vi "Error Control.vi"(4 "Command":T1, 5 "error in (no error)":errorcluster, 8 "Source":string) -> (0 "error out":errorcluster)   [LabVIEW 2020]
doc: "[Ver 1.00]\nREUSEABLE COMPONENT\nDESCRIPTION\nReuseable Component\nDisplays or logs errors. \n\nCOMMANDS\nNo Command - Error :Throw the error dialog.\nSet to Dev Mode : This should be set first, when Set Error is called the dialog will be displayed. \nSet to Released Mode : This should be set first, when Set Error is called the error will be quietly filed away.\nSet Error : Throw or Log an error.\nLog Error : Log an error regardless of Mode.\nThrow Error : Throw dialog regardless of Mode.\nLog & Throw Error : Do both regardless of Mode.\n\nERROR HANDLING\nWill throw an error if No Command is set\n\n---------------------------------------------------------\nVERSION CONTROL\n1.00 New version SSDC 14/3/2000"
uses:
  Controls/DisplayQCommand.ctl
  Error/ErrorMessage.ctl
  ErrorCommand.ctl
panel:
  # "Input"
  # "Output"
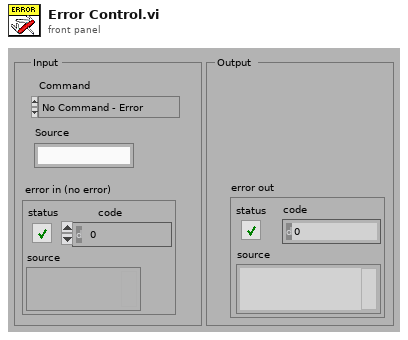
[diagram p1: front panel]
types:
  T1 = typedef "ErrorCommand.ctl" = enum16{"No Command - Error", "Set to Dev Mode", "Set To Released Mode", "Set Error", "Log Error", "Throw Error", "Log & Throw Error", "Set Error Timed"}
  T2 = typedef "ErrorMessage.ctl" = enum16{"No Message - Ignore", "Display Message", "Stop"}
  T3 = typedef "DisplayQCommand.ctl" = enum16{"No Command - Error", "Initialise", "Get Q Reference", "Add Item to Bottom", "Add Item to Top", "Flush Q", "Dequeue", "Peek Next Element", "Close"}
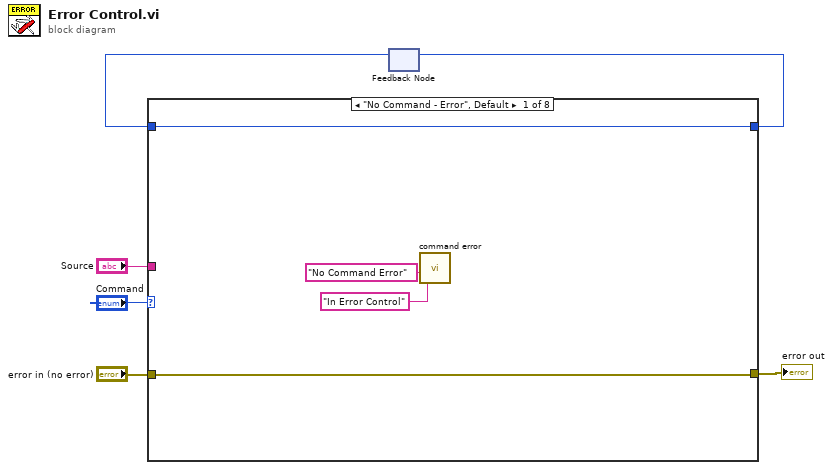
[diagram p0: block diagram]
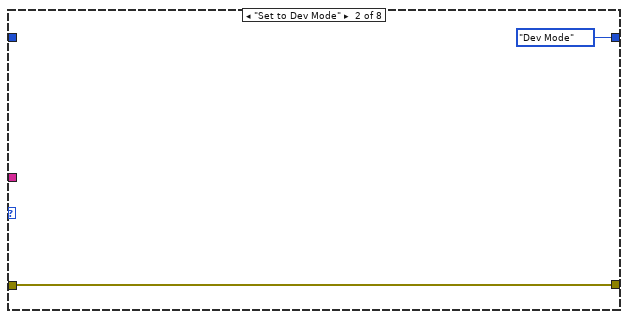
[diagram p2: hidden frame]
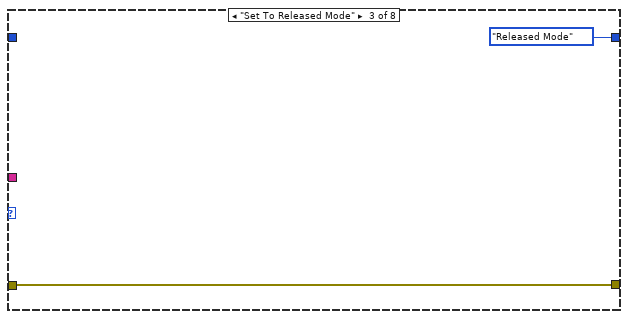
[diagram p3: hidden frame]
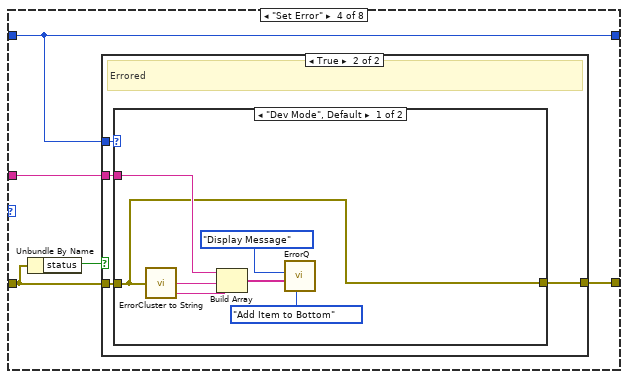
[diagram p4: hidden frame]
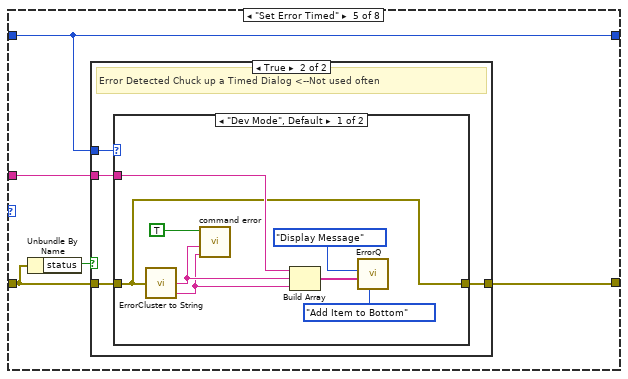
[diagram p7: hidden frame]
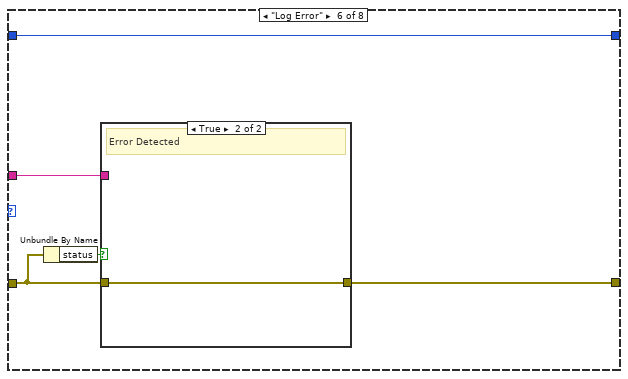
[diagram p10: hidden frame]
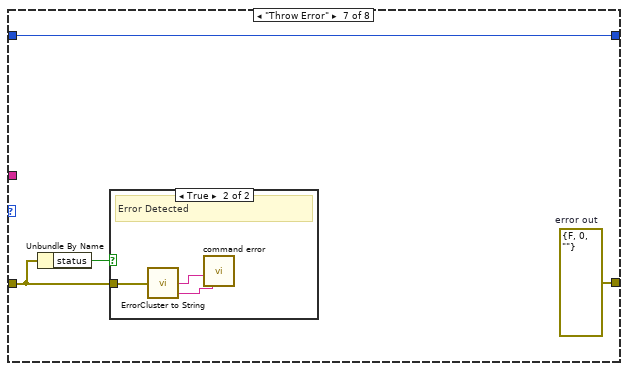
[diagram p12: hidden frame]
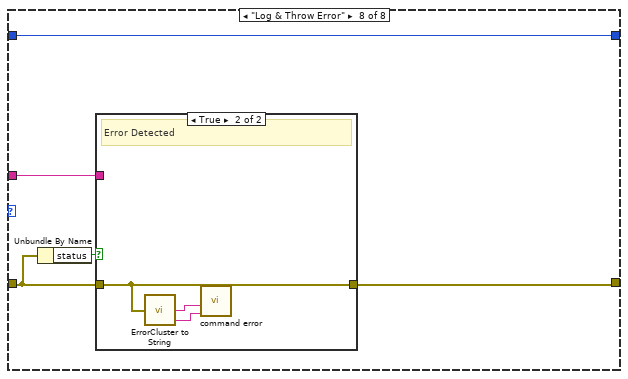
[diagram p14: hidden frame]
diagram:
  n1 = feedback #1() -> (w2:enum16{"Dev Mode", "Released Mode"})  [unwired: 1 in]
  n2 = case shown="\"No Command - Error\", Default" "Command" {
    tunnel: [w10 enum16{"Dev Mode", "Released Mode"}."Dev Mode" enum16{"Dev Mode", "Released Mode"}."Released Mode" w19 w37 w56 w62 w70] -> w3
    tunnel: w2 -> [w10 _ _ w19 w37 w56 w62 w70]
    tunnel: "error in (no error)" -> [w7 w11 w13 w18 w36 w54 w60 w68]
    tunnel: "Source" -> [_ _ _ w16 w33 w52 _ w67]
    tunnel: [w7 w11 w13 w15 w34 w53 w59 w66] -> w1
    frame "No Command - Error", Default {
      n3 = call "command error.vi"("Error Details"="In Error Control", "Comment"="No Command Error") -> ()  [unwired: 6 in]
    }
    frame "Set to Dev Mode" {
    }
    frame "Set To Released Mode" {
    }
    frame "Set Error" {
      n4 = Unbundle By Name(w18) -> ("status"=w17:bool)
      n5 = case shown="True" w17 {
        tunnel: w19 -> [_ w24]
        tunnel: w18 -> [w20 w23]
        tunnel: w16 -> [_ w22]
        tunnel: [w20 w21] -> w15
        frame False {
          # "No Error Ignore"
        }
        frame True {
          # "Errored"
          n6 = case shown="\"Dev Mode\", Default" w24 {
            tunnel: w23 -> [w25 w32]
            tunnel: w22 -> [w26 _]
            tunnel: [w25 w32] -> w21
            frame "Dev Mode", Default {
              n7 = call "ErrorCluster to String.vi"("error in (no error)"=w25) -> ("ErrorMSG"=w29:string, "String"=w28:string)  [unwired: 3 in]
              n8 = Build Array(w26, w28, w29) -> (w27:string[])
              n9 = call "ErrorQ.vi"("command"=DisplayQCommand."Add Item to Bottom", "DataIn"=w27, "ErrorMessage"=ErrorMessage."Display Message") -> ()  [unwired: 2 in, 4 out]
            }
            frame "Released Mode" {
            }
          }
        }
      }
    }
    frame "Set Error Timed" {
      n10 = Unbundle By Name(w36) -> ("status"=w35:bool)
      n11 = case shown="True" w35 {
        tunnel: w37 -> [_ w42]
        tunnel: w36 -> [w38 w41]
        tunnel: [w38 w40] -> w34
        tunnel: w33 -> [_ w39]
        frame False {
          # "No Error"
        }
        frame True {
          # "Error Detected Chuck up a Timed Dialog <--Not used often"
          n12 = case shown="\"Dev Mode\", Default" w42 {
            tunnel: w41 -> [w43 w51]
            tunnel: [w43 w51] -> w40
            tunnel: w39 -> [w46 _]
            frame "Dev Mode", Default {
              n13 = call "ErrorCluster to String.vi"("error in (no error)"=w43) -> ("ErrorMSG"=w44:string, "String"=w45:string)  [unwired: 3 in]
              n14 = call "command error.vi"("Error Details"=w44, "Comment"=w45, "5 Sec Countdown"=TRUE) -> ()  [unwired: 5 in]
              n15 = Build Array(w46, w45, w44) -> (w47:string[])
              n16 = call "ErrorQ.vi"("command"=DisplayQCommand."Add Item to Bottom", "DataIn"=w47, "ErrorMessage"=ErrorMessage."Display Message") -> ()  [unwired: 2 in, 4 out]
            }
            frame "Released Mode" {
            }
          }
        }
      }
    }
    frame "Log Error" {
      n17 = Unbundle By Name(w54) -> ("status"=w55:bool)
      n18 = case shown="True" w55 {
        tunnel: w54 -> [w57 w58]
        tunnel: [w57 w58] -> w53
        tunnel: w52 -> [_ _]
        frame False {
          # "No Error Ignore"
        }
        frame True {
          # "Error Detected"
        }
      }
    }
    frame "Throw Error" {
      w59 = errorcluster {"status"=FALSE, "code"=0, "source"=""}  # error out
      n19 = Unbundle By Name(w60) -> ("status"=w61:bool)
      n20 = case shown="True" w61 {
        tunnel: w60 -> [_ w65]
        frame False {
          # "No Error Detected"
        }
        frame True {
          # "Error Detected"
          n21 = call "ErrorCluster to String.vi"("error in (no error)"=w65) -> ("ErrorMSG"=w63:string, "String"=w64:string)  [unwired: 3 in]
          n22 = call "command error.vi"("Error Details"=w63, "Comment"=w64) -> ()  [unwired: 6 in]
        }
      }
    }
    frame "Log & Throw Error" {
      n23 = Unbundle By Name(w68) -> ("status"=w69:bool)
      n24 = case shown="True" w69 {
        tunnel: w68 -> [w71 w72]
        tunnel: w67 -> [_ _]
        tunnel: [w71 w72] -> w66
        frame False {
          # "No Error Detected"
        }
        frame True {
          # "Error Detected"
          n25 = call "ErrorCluster to String.vi"("error in (no error)"=w72) -> ("ErrorMSG"=w73:string, "String"=w74:string)  [unwired: 3 in]
          n26 = call "command error.vi"("Error Details"=w73, "Comment"=w74) -> ()  [unwired: 6 in]
        }
      }
    }
  }
  "error out" <- w1
  n27 = feedback-in #1(w3) -> ()
